vi "Write.vi"(8 "error in (no error)":errorcluster, 10 "Array":string[](array[string]), 11 "Abs_String in":refnum<class "Abs_String 1D.lvclass">) -> (0 "error out":errorcluster, 3 "Abs_String out":refnum<class "Abs_String 1D.lvclass">)   [LabVIEW 2021, in "Abs_String 1D.lvclass"]
uses:
  Abs_String 1D.lvclass
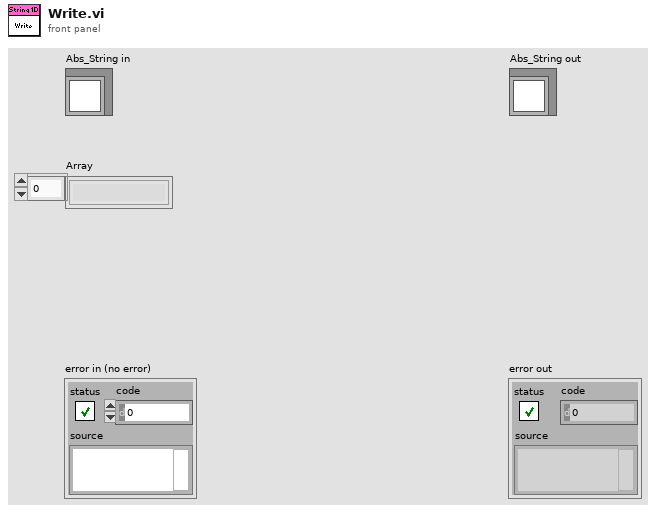
[diagram p1: front panel]
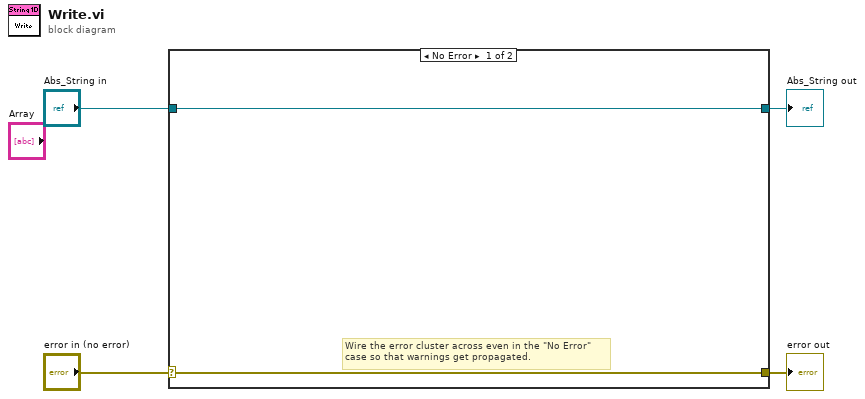
[diagram p0: block diagram]
diagram:
  n1 = case shown="No Error" "error in (no error)" {
    selector: "error in (no error)" -> [w5 w8]
    tunnel: [w5 w8] -> w3
    tunnel: [w6 w7] -> w1
    tunnel: "Abs_String in" -> [w6 w7]
    frame No Error {
      # "Wire the error cluster across even in the \"No Error\"\ncase so that warnings get propagated."
    }
    frame Error {
    }
  }
  "error out" <- w3
  "Abs_String out" <- w1
